vi "Initialise Raw Data Network Stream).vi"(8 "error in (no error)":errorcluster) -> (0 "error out":errorcluster, 3 "Refnum out":refnum<k21>)   [LabVIEW 2017]
uses:
  <vilib>/dex/Stream Element Allocation Mode.ctl
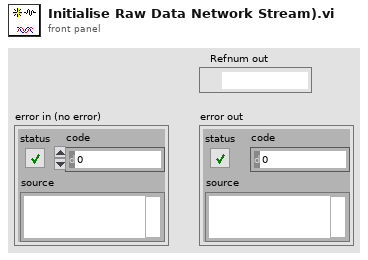
[diagram p1: front panel]
types:
  T1 = typedef "Stream Element Allocation Mode.ctl" = u32
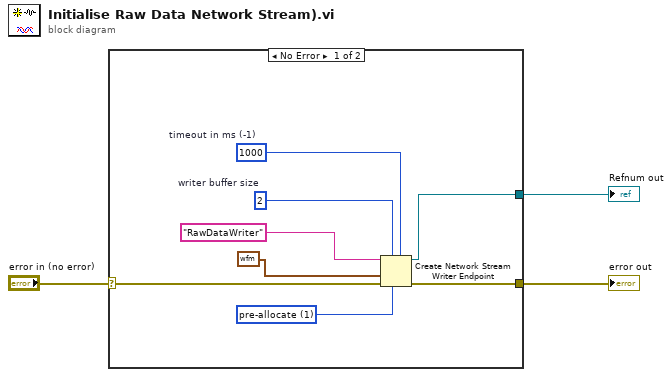
[diagram p0: block diagram]
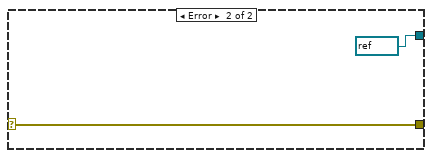
[diagram p2: hidden frame]
diagram:
  n1 = case shown="No Error" "error in (no error)" {
    selector: "error in (no error)" -> [w7 w13]
    tunnel: [w6 w13] -> w1
    tunnel: [w5 refnum<k21> refnum ("writer name")] -> w3
    frame No Error {
      w8 = T1 1 items=["allocate as needed", "pre-allocate"] ("element allocation mode")
      w9 = 1000  # timeout in ms (-1)
      w10 = 2  # writer buffer size
      n2 = Create Network Stream Writer Endpoint(5:w9, 6:w8, 7:w10, 8:w7, 9:waveform(u8) {"t0"=timestamp(0 s since 1904-01-01), "dt"=1.0, "Y"=[]} ("output waveform"), 11:"RawDataWriter" ("writer name")) -> (0:w6:errorcluster, 3:w5:refnum<k21>)  [unwired: 1 in]
    }
    frame Error {
    }
  }
  "Refnum out" <- w3
  "error out" <- w1
